vi "CRC_16CITT_A.vi"(6 "Error In":errorcluster, 7 "DATA PACKET":string) -> (0 "Error Out":errorcluster, 1 "DATA PACKET+CRC":string, 2 "CRC out":u16 format="%x")   [LabVIEW 2019]
doc: "Данная VI предназначена для расчета CRC-16CITT, которая используется для стандарта ISO/IEC 14443 Type A и ISO/IEC 18092 Felica."
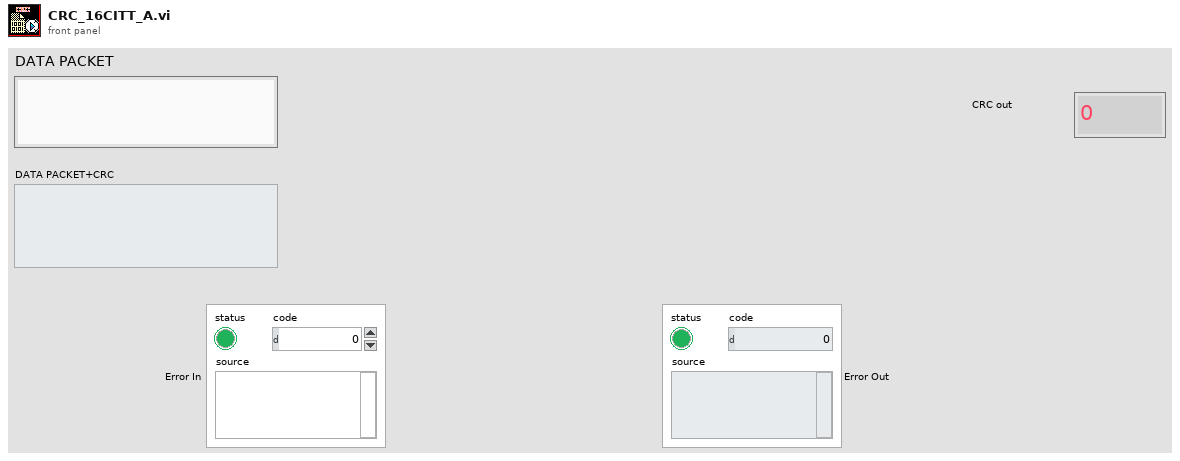
[diagram p1: front panel]
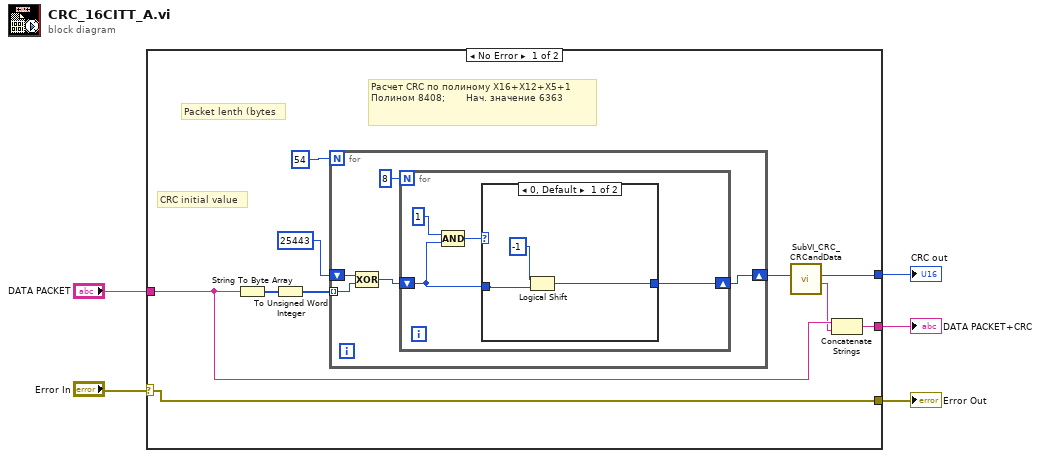
[diagram p0: block diagram]
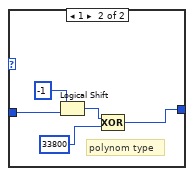
[diagram p2: hidden frame]
diagram:
  n1 = case shown="No Error" "Error In" {
    selector: "Error In" -> [w9 w34]
    tunnel: [w6 _] -> w5
    tunnel: "DATA PACKET" -> [w11 w33]
    tunnel: [w10 w33] -> w3
    tunnel: [w9 w34] -> w1
    frame No Error {
      # "Packet lenth (bytes"
      # "CRC initial value"
      # "Расчет CRC по полиному X16+X12+X5+1\nПолином 8408;       Нач. значение 6363"
      n2 = String To Byte Array(string=w11) -> (unsigned byte array=w13:u8[])
      n3 = To Unsigned Word Integer(number=w13) -> (unsigned 16bit integer=w12:u16[])
      n4 = for {
        N: 54 -> [_]
        shift-right: [w16] -> w8
        shift-left: u16 25443 -> [w18]
        tunnel: w12 -> [w19] mode=indexing
        n5 = Compound Arithmetic op=XOR(w18, w19) -> (w17:u32)
        n6 = for {
          N: 8 -> [_]
          shift-right: [w23] -> w16
          shift-left: w17 -> [w22]
          n7 = Compound Arithmetic op=AND(u16 1, w22) -> (w21:u32)
          n8 = case shown="0, Default" w21 {
            tunnel: [w25 w28] -> w23
            tunnel: w22 -> [w26 w31]
            frame 0, Default {
              n9 = Logical Shift(y=i16 -1, x=w26) -> (x << y=w25:u32)
            }
            frame 1 {
              # "polynom type"
              n10 = Logical Shift(y=i16 -1, x=w31) -> (x << y=w30:u32)
              n11 = Compound Arithmetic op=XOR(w30, u32 33800) -> (w28:u32)
            }
          }
        }
      }
      n12 = call "SubVI_CRC_CRCandData.vi"("CRC in"=w8) -> ("CRC out(str)"=w7:string, "CRC out"=w6:u32)  [unwired: 8 in, 1 out]
      n13 = Concatenate Strings(w11, w7) -> (w10:string)
    }
    frame Error {
    }
  }
  "CRC out" <- w5
  "DATA PACKET+CRC" <- w3
  "Error Out" <- w1
